vi "Pluma-VI.vi"(9 "Parar el funcionamiento":bool, 10 "Pluma":T1) -> (1 "Stop value":bool)   [LabVIEW 2024]
doc: "Este VI se encarga de simular la pluma de una caseta de estacionamiento, toma dos casos, abrir y cerrar, en caso de que se desee abrir la pluma se mueve 90° hacia la derecha, y en caso de cerrar se mueve la pluma 90° hacia la izquierda.\n\n03/10/2024\n\nRoberto Gomez Cruz, Ivan Nieto Guerrero y David Alejandro Zarazua Martinez (yucateco)"
uses:
  Abrir_cerrar pluma.ctl
  <vilib>/DAQmx/write.llb/DAQmx Write (Digital 1D Bool NChan 1Samp 1Line).vi
  <vilib>/DAQmx/miscellaneous.llb/DAQmx Fill In Error Info.vi
panel:
  # "Control de estacionamiento"
  # "Caseta"
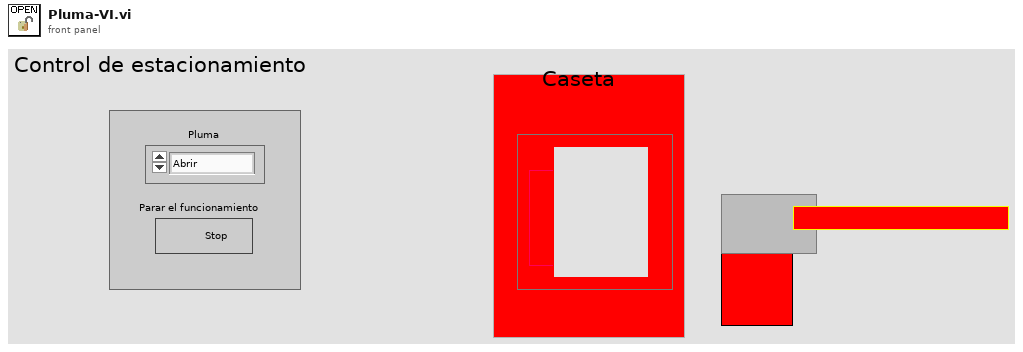
[diagram p1: front panel]
types:
  T1 = typedef "Abrir_cerrar pluma.ctl" = enum16{"Abrir", "Cerrar"}
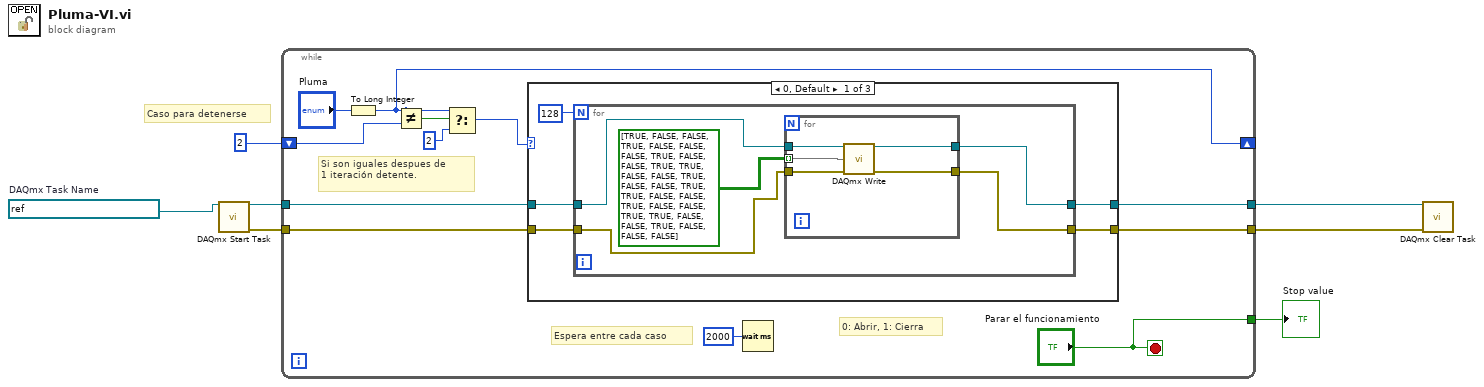
[diagram p0: block diagram]
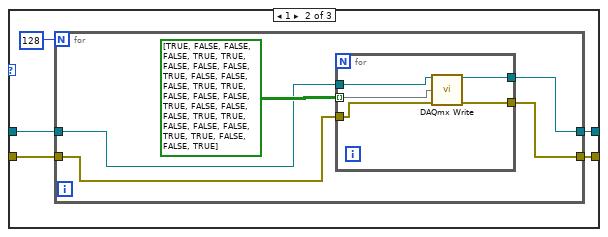
[diagram p2: hidden frame]
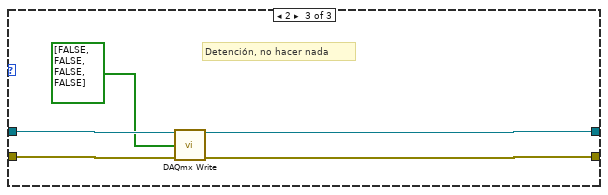
[diagram p3: hidden frame]
diagram:
  w3 = refnum<k21> "MyDigitalOutTask_TEST"  # DAQmx Task Name
  # "Caso para detenerse"
  n1 = call <vilib>:"DAQmx Start Task.vi"("task/channels in"=w3) -> ("task out"=w7:refnum<k21>, "error out"=w6:errorcluster)  [unwired: 13 in]
  n2 = while {
    tunnel: w7 -> [w19]
    tunnel: w6 -> [w18]
    shift-right: [w13] -> _
    shift-left: 2 -> [w16]
    tunnel: [w11] -> w4
    tunnel: [w10] -> w2
    tunnel: ["Parar el funcionamiento"] -> w1
    stop <- "Parar el funcionamiento" stop-if-true
    # "Espera entre cada caso"
    # "Si son iguales despues de\n1 iteración detente."
    # "0: Abrir, 1: Cierra"
    n3 = To Long Integer(number="Pluma") -> (32bit integer=w13:i32)
    n4 = Not Equal?(x=w13, y=w16) -> (x != y?=w15:bool)
    n5 = Select(t=w13, s=w15, f=2) -> (s? t:f=w14:i32)
    n6 = case shown="0, Default" w14 {
      tunnel: w19 -> [w23 w39 w52]
      tunnel: w18 -> [w22 w38 w51]
      tunnel: [w20 w35 w54] -> w10
      tunnel: [w21 w36 w53] -> w11
      frame 0, Default {
        n7 = for {
          N: 128 -> [_]
          tunnel: w23 -> [w26]
          tunnel: w22 -> [w25]
          tunnel: [w29] -> w20
          tunnel: [w28] -> w21
          n8 = for {
            tunnel: [w34] -> w29
            tunnel: [w33] -> w28
            tunnel: bool[][] [[TRUE, FALSE, FALSE, TRUE], [FALSE, FALSE, FALSE, TRUE], [FALSE, FALSE, TRUE, TRUE], [FALSE, FALSE, TRUE, FALSE], [FALSE, TRUE, TRUE, FALSE], [FALSE, TRUE, FALSE, FALSE], [TRUE, TRUE, FALSE, FALSE], [TRUE, FALSE, FALSE, FALSE]] -> [w32] mode=indexing
            tunnel: w26 -> [w31]
            tunnel: w25 -> [w30]
            n9 = call-poly <vilib>:"DAQmx Write.vi"("task/channels in"=w31, "data"=w32, "error in"=w30) -> ("task out"=w34:refnum<k21>, "error out"=w33:errorcluster)  [unwired: 10 in, 1 out]
          }
        }
      }
      frame 1 {
        n10 = for {
          N: 128 -> [_]
          tunnel: w39 -> [w42]
          tunnel: w38 -> [w43]
          tunnel: [w41] -> w36
          tunnel: [w40] -> w35
          n11 = for {
            tunnel: bool[][] [[TRUE, FALSE, FALSE, FALSE], [TRUE, TRUE, FALSE, FALSE], [FALSE, TRUE, FALSE, FALSE], [FALSE, TRUE, TRUE, FALSE], [FALSE, FALSE, TRUE, FALSE], [FALSE, FALSE, TRUE, TRUE], [FALSE, FALSE, FALSE, TRUE], [TRUE, FALSE, FALSE, TRUE]] -> [w49] mode=indexing
            tunnel: w43 -> [w48]
            tunnel: w42 -> [w47]
            tunnel: [w46] -> w40
            tunnel: [w45] -> w41
            n12 = call-poly <vilib>:"DAQmx Write.vi"("task/channels in"=w47, "data"=w49, "error in"=w48) -> ("task out"=w46:refnum<k21>, "error out"=w45:errorcluster)  [unwired: 10 in, 1 out]
          }
        }
      }
      frame 2 {
        # "Detención, no hacer nada"
        n13 = call-poly <vilib>:"DAQmx Write.vi"("task/channels in"=w52, "data"=bool[] [FALSE, FALSE, FALSE, FALSE], "error in"=w51) -> ("task out"=w54:refnum<k21>, "error out"=w53:errorcluster)  [unwired: 10 in, 1 out]
      }
    }
    n14 = Wait (ms)(milliseconds to wait=u32 2000) -> ()  [unwired: 1 out]
  }
  "Stop value" <- w1
  n15 = call <vilib>:"DAQmx Clear Task.vi"("task in"=w2, "error in"=w4) -> ()  [unwired: 13 in, 1 out]
